vi "Setup For Ping.vi"(5 "TTL (U8)":u8=128, 6 "Timeout (ms)":i32=1000, 7 "Host to Ping":string, 8 "Error In":errorcluster) -> (0 "Error Out":errorcluster, 2 "Resolved IP":u32 format="%x", 3 "Socket Out":u32 format="%x")   [LabVIEW 2018]
panel:
  in  "Case Constant\n(See Context Help)":bool
  out "Tx Timeout Readback":i32
  out "Rx Timeout Readback":i32
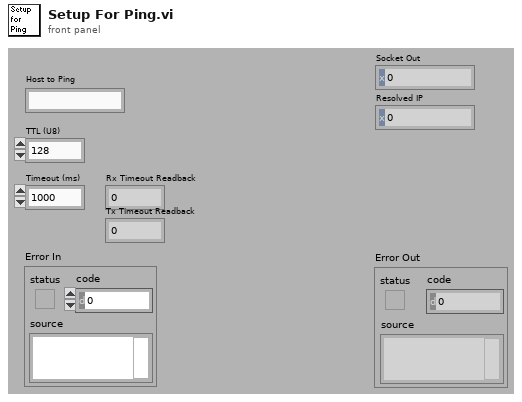
[diagram p1: front panel]
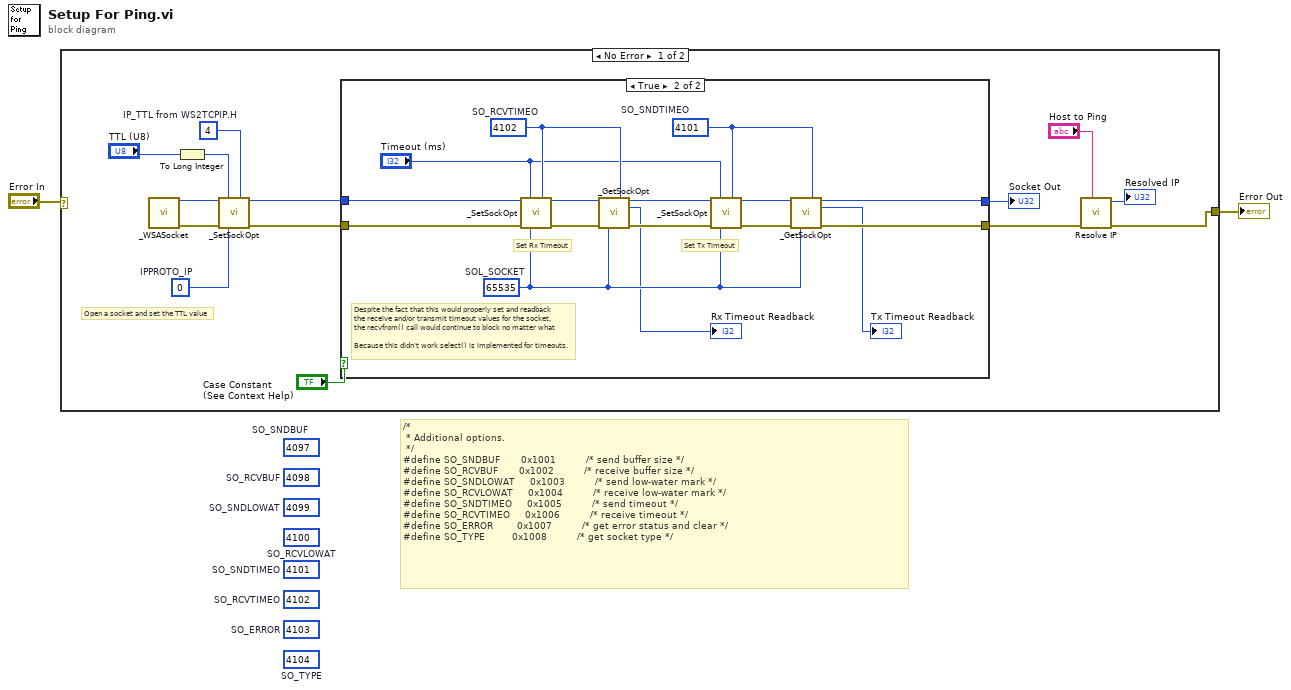
[diagram p0: block diagram]
diagram:
  (unwired) 4097  # SO_SNDBUF
  (unwired) 4098  # SO_RCVBUF
  (unwired) 4099  # SO_SNDLOWAT
  (unwired) 4100  # SO_RCVLOWAT
  (unwired) 4101  # SO_SNDTIMEO
  (unwired) 4102  # SO_RCVTIMEO
  (unwired) 4103  # SO_ERROR
  (unwired) 4104  # SO_TYPE
  # "/*\n * Additional options.\n */\n#define SO_SNDBUF       0x1001          /* send buffer size */\n#define SO_RCVBUF       0x1002          /* receive buffer size */\n#define SO_SNDLOWAT     0x1003          /* send low-water mark */\n#define SO_RCVLOWAT     0x1004          /* receive low-water mark */\n#define SO_SNDTIMEO     0x1005          /* send timeout */\n#define SO_RCVTIMEO     0x1006          /* receive timeout */\n#define SO_ERROR        0x1007          /* get error status and clear */\n#define SO_TYPE         0x1008          /* get socket type */"
  n1 = case shown="No Error" "Error In" {
    selector: "Error In" -> [_ w35]
    tunnel: [w13 w35] -> w1
    frame No Error {
      w9 = 0  # IPPROTO_IP
      w5 = 4  # IP_TTL from WS2TCPIP.H
      # "Open a socket and set the TTL value"
      n2 = call "_WSASocket.vi"() -> ("Error Out"=w16:errorcluster, "Socket"=w6:u32)  [unwired: 10 in]
      n3 = To Long Integer(number="TTL (U8)") -> (32bit integer=w4:i32)
      n4 = call "_SetSockOpt.vi"("Socket"=w6, "Option (I32)"=w4, "OptionName"=w5, "Error In"=w16, "Level"=w9) -> ("Socket Out"=w7:u32, "Error Out"=w12:errorcluster)  [unwired: 8 in, 1 out]
      n5 = case shown="True" "Case Constant\n(See Context Help)" {
        tunnel: w12 -> [w18 w34]
        tunnel: [w18 w25] -> w11
        tunnel: [w17 w24] -> w10
        tunnel: w7 -> [w17 w23]
        frame False {
        }
        frame True {
          w19 = 4101  # SO_SNDTIMEO
          w26 = 65535  # SOL_SOCKET
          w29 = 4102  # SO_RCVTIMEO
          # "Despite the fact that this would properly set and readback\nthe receive and/or transmit timeout values for the socket,\nthe recvfrom() call would continue to block no matter what\n\nBecause this didn't work select() is implemented for timeouts."
          # "Set Rx Timeout"
          # "Set Tx Timeout"
          n6 = call "_SetSockOpt.vi"("Socket"=w23, "Option (I32)"="Timeout (ms)", "OptionName"=w29, "Error In"=w34, "Level"=w26) -> ("Socket Out"=w33:u32, "Error Out"=w32:errorcluster)  [unwired: 8 in, 1 out]
          n7 = call "_GetSockOpt.vi"("Socket"=w33, "OptionName"=w29, "Error In"=w32, "Level"=w26) -> ("Socket Out"=w31:u32, "Value (I32)"=→"Rx Timeout Readback":i32, "Error Out"=w30:errorcluster)  [unwired: 7 in, 2 out]
          n8 = call "_SetSockOpt.vi"("Socket"=w31, "Option (I32)"="Timeout (ms)", "OptionName"=w19, "Error In"=w30, "Level"=w26) -> ("Socket Out"=w28:u32, "Error Out"=w27:errorcluster)  [unwired: 8 in, 1 out]
          n9 = call "_GetSockOpt.vi"("Socket"=w28, "OptionName"=w19, "Error In"=w27, "Level"=w26) -> ("Socket Out"=w24:u32, "Value (I32)"=→"Tx Timeout Readback":i32, "Error Out"=w25:errorcluster)  [unwired: 7 in, 2 out]
        }
      }
      "Socket Out" <- w10
      n10 = call "Resolve IP.vi"("Host to Ping"="Host to Ping", "Error In"=w11) -> ("Error Out"=w13:errorcluster, "Resolved IP"=→"Resolved IP":u32)  [unwired: 8 in]
    }
    frame Error {
    }
  }
  "Error Out" <- w1
